vi "CRC32.vi"(8 "error in (no error)":errorcluster, 11 "FILE IN":path) -> (0 "error out":errorcluster, 2 "CRC32Value":u32 format="%x", 3 "FILE OUT":path)   [LabVIEW 2019]
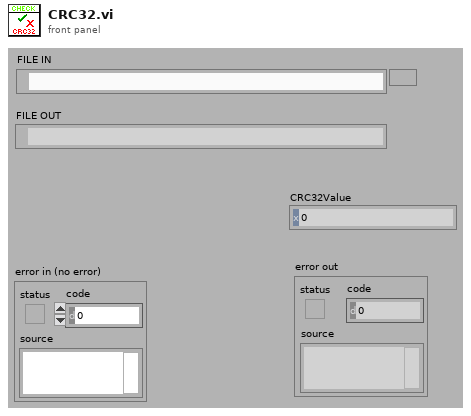
[diagram p1: front panel]
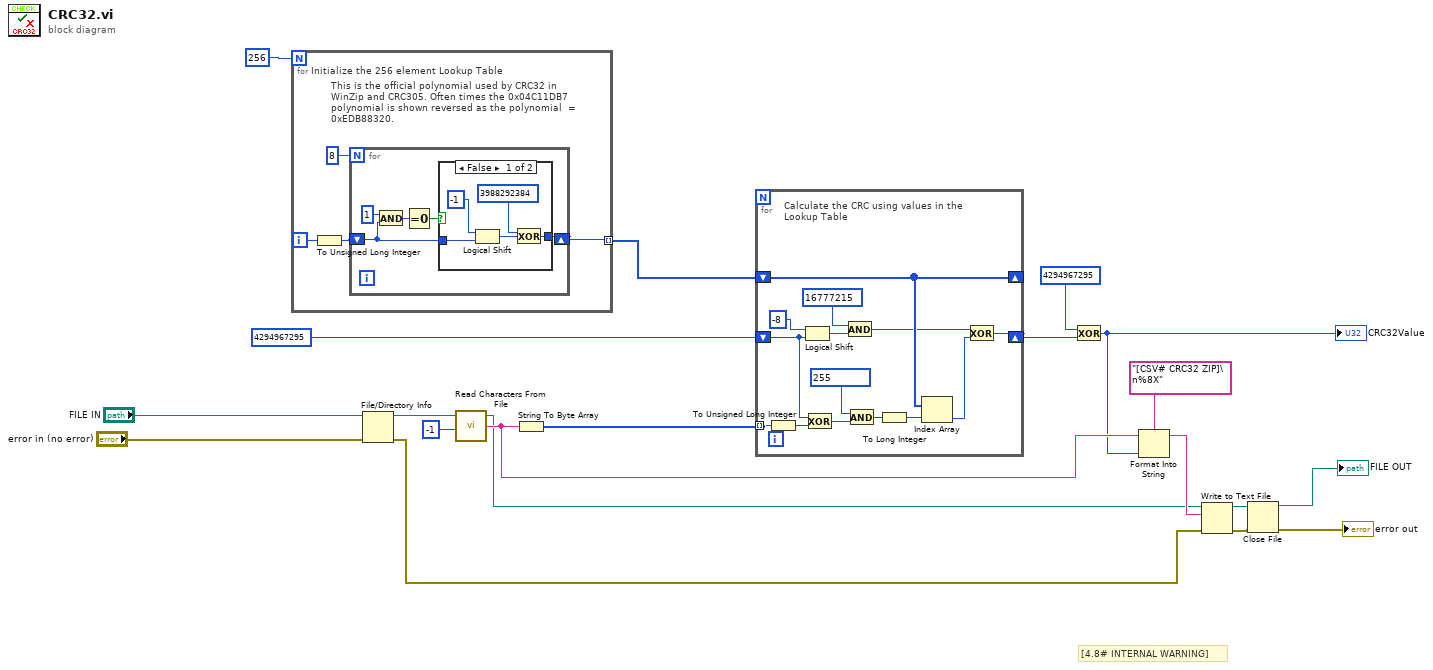
[diagram p0: block diagram]
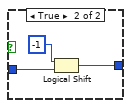
[diagram p2: hidden frame]
diagram:
  # "[4.8# INTERNAL WARNING]"
  n1 = for {
    N: 256 -> [_]
    tunnel: [w23] -> w13 mode=indexing
    i -> [w22]
    # "This is the official polynomial used by CRC32 in WinZip and CRC305. Often times the 0x04C11DB7 polynomial is shown reversed as the polynomial  = 0xEDB88320."
    # "Initialize the 256 element Lookup Table"
    n2 = To Unsigned Long Integer(number=w22) -> (unsigned 32bit integer=w21:u32)
    n3 = for {
      N: 8 -> [_]
      shift-right: [w29] -> w23
      shift-left: w21 -> [w28]
      n4 = And(x=u32 1, y=w28) -> (x .and. y?=w27:u32)
      n5 = Equal To 0?(x=w27) -> (x = 0?=w25:bool)
      n6 = case shown="False" w25 {
        tunnel: w28 -> [w34 w37]
        tunnel: [w30 w35] -> w29
        frame False {
          n7 = Logical Shift(y=-1, x=w34) -> (x << y=w32:u32)
          n8 = Exclusive Or(1:w32, 2:u32 3988292384) -> (0:w30:u32)
        }
        frame True {
          n9 = Logical Shift(y=-1, x=w37) -> (x << y=w35:u32)
        }
      }
    }
  }
  n10 = File/Directory Info(path="FILE IN", error in="error in (no error)") -> (path out=w16:path, error out=w11:errorcluster)  [unwired: 5 out]
  n11 = call <vilib>:"Read Characters From File.vi"("file path (dialog if empty)"=w16, "number of characters (all:-1)"=-1) -> ("new file path (NotAPath if cancelled)"=w1:path, "character string"=w5:string)  [unwired: 4 in, 2 out]
  n12 = String To Byte Array(string=w5) -> (unsigned byte array=w19:u8[])
  n13 = for {
    tunnel: w19 -> [w51] mode=indexing
    shift-right: [w44] -> w15
    shift-left: u32 4294967295 ("CRCBuffer") -> [w40]
    shift-right: [w43] -> _
    shift-left: w13 -> [w43]
    # "Calculate the CRC using values in the Lookup Table"
    n14 = To Unsigned Long Integer(number=w51) -> (unsigned 32bit integer=w50:u32)
    n15 = Logical Shift(y=-8, x=w40) -> (x << y=w45:u32)
    n16 = Exclusive Or(1:w50, 2:w40) -> (0:w48:u32)
    n17 = And(x=u32 16777215, y=w45) -> (x .and. y?=w42:u32)
    n18 = And(x=u32 255, y=w48) -> (x .and. y?=w39:u32)
    n19 = To Long Integer(number=w39) -> (32bit integer=w47:i32)
    n20 = Index Array(array=w43, index=w47) -> (element=w46:u32)
    n21 = Exclusive Or(1:w46, 2:w42) -> (0:w44:u32)
  }
  n22 = Exclusive Or(1:w15, 2:u32 4294967295) -> (0:w3:u32)
  "CRC32Value" <- w3
  n23 = Format Into String(format string="[CSV# CRC32 ZIP]\n%8X", initial string=w5, w3) -> (resulting string=w2:string)  [unwired: 1 in, 1 out]
  n24 = Write to Text File(file (use dialog)=w1, text=w2, error in=w11) -> (refnum out=w10:refnum<file>, error out=w9:errorcluster)  [unwired: 1 in, 1 out]
  n25 = Close File(refnum=w10, error in=w9) -> (path=→"FILE OUT":path, error out=→"error out":errorcluster)
